vi "Cluster Group Names.vi"(8 "error in (no error)":errorcluster, 11 "Historian Module in":refnum<class "Historian Module.lvclass">) -> (0 "error out":errorcluster, 2 "Group Names":string[](array[string]), 3 "Historian Module out":refnum<class "Historian Module.lvclass">)   [LabVIEW 2020, in "VolatusHistorian.lvlib" / "Historian Module.lvclass"]
uses:
  Historian Module.lvclass
  C:/dev/lv20CE/relink/lv-volatus/Volatus/Module/Module.lvclass
  VolatusConfig/Meta Type.ctl
  Volatus/Module/Module.lvclass/Module.ctl
  VolatusConfig/VolatusConfigElement/VolatusConfigElement.lvclass/VolatusConfigElement.ctl
  VolatusConfig/VolatusConfigElement/Element.vi
  lv-cdm/CDM-Config/Config Element/Owner.vi
  lv-cdm/CDM-Config/Config Manager/Lookup Descendant.vi
  lv-cdm/CDM-Config/Config Filter/Config Lookup.lvclass
  Historian Module.lvclass/Historian Module.ctl
  Volatus/Module/Module.lvclass
  VolatusConfig/VolatusConfigElement/VolatusConfigElement.lvclass
  VolatusConfig/VolatusConfig.lvlib
  lv-cdm/CDM-Config/Config Element/Config Element.lvclass
  C:/dev/lv20CE/relink/lv-volatus/VolatusHistorian/Historian Module/Historian Module.lvclass
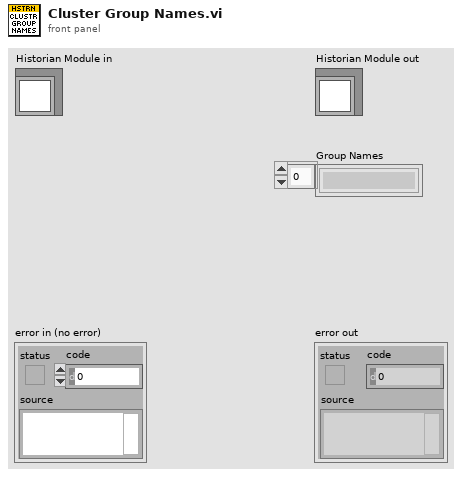
[diagram p1: front panel]
types:
  T1 = typedef "VolatusConfig.lvlib/Meta Type.ctl" = enum16{"UNKNOWN", "VL_System", "VL_Cluster", "VL_Node", "VL_Task", "VL_Group", "VL_Channel", "VL_Task_List", "VL_Scaling", "VL_Sensor", "VL_Sensor_List", "VL_Scale"}
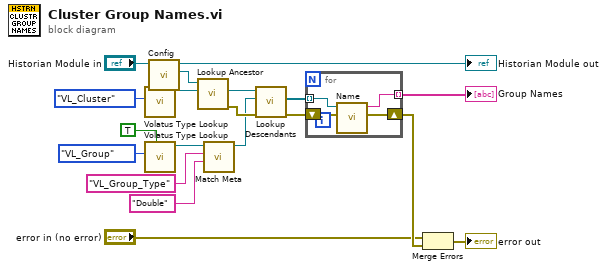
[diagram p0: block diagram]
diagram:
  n1 = call "Volatus Type Lookup.vi"("Meta Type"=Meta_Type."VL_Cluster") -> ("Config Lookup out"=w16:refnum<class "Config Lookup.lvclass">)  [unwired: 9 in, 1 out]
  n2 = call "Volatus Type Lookup.vi"("Don't Recurse Past Match (F)"=TRUE, "Meta Type"=Meta_Type."VL_Group") -> ("Config Lookup out"=w12:refnum<class "Config Lookup.lvclass">)  [unwired: 8 in, 1 out]
  n3 = call "Config.vi"("Module in"="Historian Module in") -> ("Config"=w17:refnum<class "VolatusConfigElement.lvclass">, "Module out"=→"Historian Module out":refnum<class "Historian Module.lvclass">)  [unwired: 9 in]
  n4 = call "Lookup Ancestor.vi"("Lookup"=w16, "VolatusConfigElement in"=w17) -> ("error out"=w19:errorcluster, "Ancestor"=w13:refnum<class "Config Element.lvclass">)  [unwired: 7 in, 1 out]
  n5 = call "Match Meta.vi"("Value (Any)"="Double" ("Name"), "Name"="VL_Group_Type", "Config Lookup (New)"=w12) -> ("Config Lookup out"=w3:refnum<class "Config Lookup.lvclass">)  [unwired: 7 in, 1 out]
  n6 = call "Lookup Descendants.vi"("error in (no error)"=w19, "Lookup"=w3, "Config Element in"=w13) -> ("error out"=w9:errorcluster, "Descendants"=w10:refnum<class "Config Element.lvclass">[])  [unwired: 6 in, 1 out]
  n7 = for {
    tunnel: w10 -> [w23] mode=indexing
    shift-right: [w21] -> w7
    shift-left: w9 -> [w22]
    tunnel: [w20] -> w8 mode=indexing
    n8 = call "Name.vi"("error in (no error)"=w22, "Config Element in"=w23) -> ("error out"=w21:errorcluster, "Name"=w20:string)  [unwired: 8 in]
  }
  "Group Names" <- w8
  n9 = Merge Errors("error in (no error)", w7) -> (→"error out":errorcluster)
